vi "Write element_1.vi"(9 "seconds since 1Jan1904":timestamp, 10 "Variant":variant, 11 "node ID":T1) -> (3 "request out":T2 {"node status" items=["Good"=0, "Uncertain"=1073741824, "Uncertain_InitialValue"=1083310080, "Uncertain_LastUsableValue"=1083179008, "Uncertain_SensorNotAccurate"=1083375616, "Uncertain_EngineeringUnitsExceeded"=1083441152, "Bad"=2147483648, "Bad_NoCommunication"=2150694912, "Bad_NotReadable"=2151284736, "Bad_NotWritable"=2151350272, "Bad_OutOfRange"=2151415808, "Bad_WaitingForInitialData"=2150760448]})   [LabVIEW 2019, in "OPC addons.lvlib"]
uses:
  OPC addons.lvlib
  <vilib>/OPCUA/controls/Write Variant Request.ctl
  <vilib>/OPCUA/controls/NodeId.ctl
  <vilib>/OPCUA/controls/Write Status.ctl
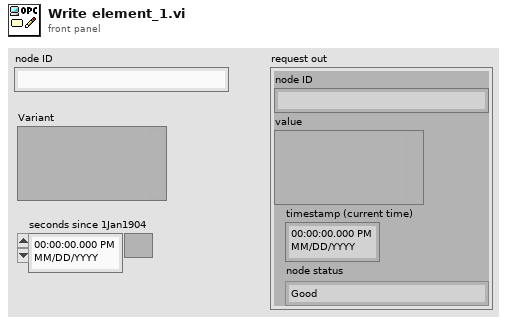
[diagram p1: front panel]
types:
  T1 = typedef "NodeId.ctl" = string
  T2 = typedef "Write Variant Request.ctl" = cluster{"node ID":T1, "value":variant, "timestamp (current time)":timestamp, "node status":T3}
  T3 = typedef "Write Status.ctl" = u32
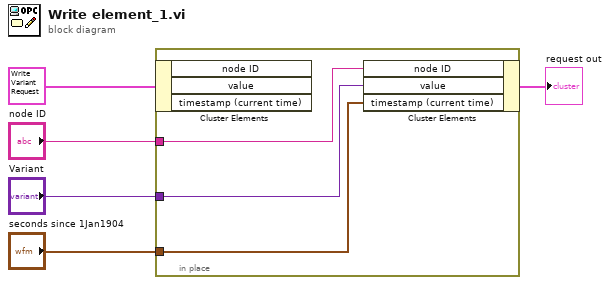
[diagram p0: block diagram]
diagram:
  n1 = in-place {
    in-place-border: "Variant" -> [w8]
    in-place-border: "seconds since 1Jan1904" -> [w7]
    in-place-border: "node ID" -> [w6]
    n2 = in-place-cluster #1(T2 {"node ID"="", "value"=variant, "timestamp (current time)"=timestamp(0 s since 1904-01-01), "node status"=0} ("request in")) -> ()  [unwired: 3 out]
    n3 = in-place-cluster #1("node ID"=w6, "value"=w8, "timestamp (current time)"=w7) -> (→"request out":T2)
  }
